vi "Column Variant.vi"(8 "error in (no error)":errorcluster, 11 "SQL Statement in":refnum<class "SQL Statement.lvclass">) -> (0 "error out":errorcluster, 2 "Variant":variant, 3 "SQL Statement out":refnum<class "SQL Statement.lvclass">)   [LabVIEW 2023, in "SQLiteSupport.lvlib" / "SQL Statement.lvclass"]
doc: "Extracts the column value as a LabVIEW Variant using the following conversion from SQLite to LabVIEW datatypes:\nNull --> Void\nInteger --> Int64\nReal --> Double\nText (UTF-8) --> String\nBlob --> String"
uses:
  SQL Statement.lvclass
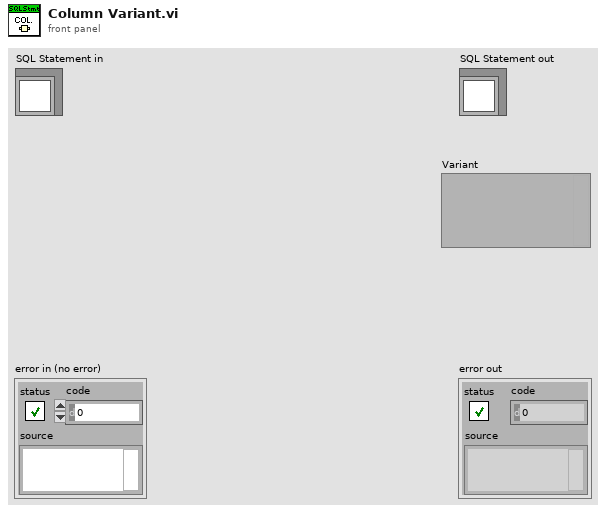
[diagram p1: front panel]
types:
  T1 = typedef "SQLiteSupport.lvlib/SQLITE Datatype.ctl" = enum32{"undefined type (0)", "SQLITE_INTEGER", "SQLITE_FLOAT", "SQLITE3_TEXT", "SQLITE_BLOB", "SQLITE_NULL", "undefined type"}
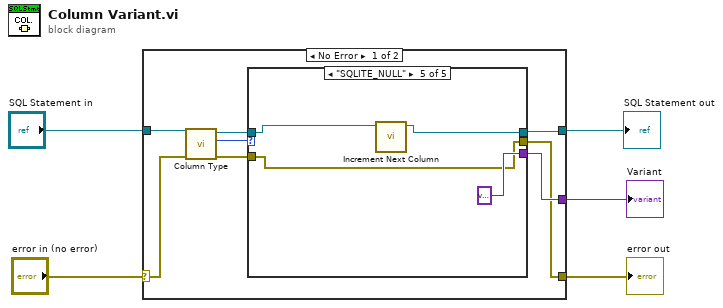
[diagram p0: block diagram]
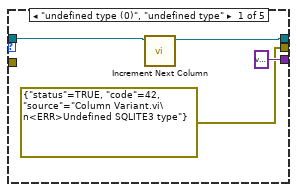
[diagram p2: hidden frame]
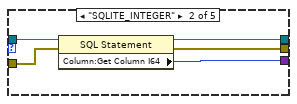
[diagram p3: hidden frame]
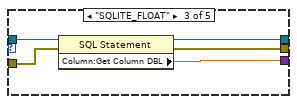
[diagram p4: hidden frame]
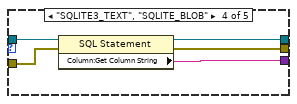
[diagram p5: hidden frame]
diagram:
  n1 = case shown="No Error" "error in (no error)" {
    selector: "error in (no error)" -> [w9 w38]
    tunnel: [w6 w38] -> w4
    tunnel: [w8 w37] -> w2
    tunnel: "SQL Statement in" -> [w13 w37]
    tunnel: [w7 _] -> w1
    frame No Error {
      n2 = call "Column Type.vi"("error in (no error)"=w9, "SQL Statement in"=w13) -> ("error out"=w10:errorcluster, "SQLite3 type"=w12:T1, "SQL Statement out"=w11:refnum<class "SQL Statement.lvclass">)  [unwired: 7 in]
      n3 = case shown="\"SQLITE_NULL\"" w12 {
        tunnel: w11 -> [w15 w22 w27 w32 w34]
        tunnel: w10 -> [_ w21 w26 w31 w35]
        tunnel: [w14 w20 w25 w30 w33] -> w8
        tunnel: [variant ("Variant") w19 w24 w29 variant ("Variant")] -> w7
        tunnel: [errorcluster {"status"=TRUE, "code"=42, "source"="Column Variant.vi\n<ERR>Undefined SQLITE3 type"} ("error out") w18 w23 w28 w35] -> w6
        frame "undefined type (0)", "undefined type" {
          n4 = call "Increment Next Column.vi"("SQL Statement in"=w15) -> ("SQL Statement out"=w14:refnum<class "SQL Statement.lvclass">)  [unwired: 10 in]
        }
        frame "SQLITE_INTEGER" {
          n5 = property class="SQL Statement"(reference=w22, error in=w21) -> (reference out=w20:refnum<class "SQL Statement.lvclass">, error out=w18:errorcluster, "Column:Get Column I64"=w19:i64)
        }
        frame "SQLITE_FLOAT" {
          n6 = property class="SQL Statement"(reference=w27, error in=w26) -> (reference out=w25:refnum<class "SQL Statement.lvclass">, error out=w23:errorcluster, "Column:Get Column DBL"=w24:dbl)
        }
        frame "SQLITE3_TEXT", "SQLITE_BLOB" {
          n7 = property class="SQL Statement"(reference=w32, error in=w31) -> (reference out=w30:refnum<class "SQL Statement.lvclass">, error out=w28:errorcluster, "Column:Get Column String"=w29:string)
        }
        frame "SQLITE_NULL" {
          n8 = call "Increment Next Column.vi"("SQL Statement in"=w34) -> ("SQL Statement out"=w33:refnum<class "SQL Statement.lvclass">)  [unwired: 10 in]
        }
      }
    }
    frame Error {
    }
  }
  "error out" <- w4
  "SQL Statement out" <- w2
  "Variant" <- w1
